vi "mqttCmdPublishTopicWrite.vi"(0 "mqttPublish in":refnum<class "mqttCmdPublish.lvclass">, 5 "topic":string, 11 "error in (no error)":errorcluster) -> (4 "mqttPublish out":refnum<class "mqttCmdPublish.lvclass">, 15 "error out":errorcluster)   [LabVIEW 2020, in "mqttCmdPublish.lvclass"]
uses:
  mqttCmdPublish.lvclass
  mqttCmdPublish.lvclass/mqttCmdPublish.ctl
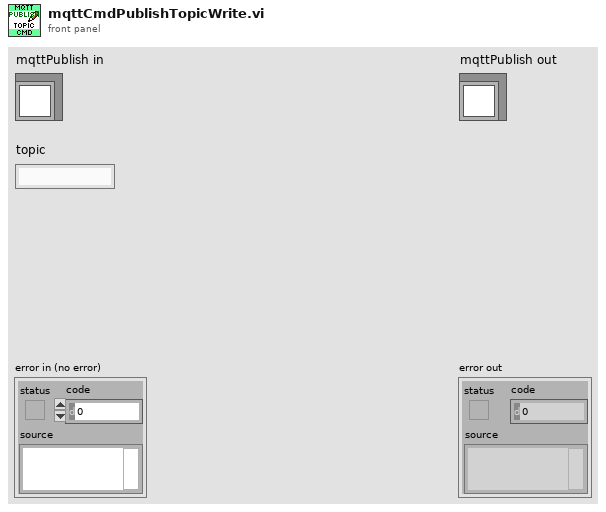
[diagram p1: front panel]
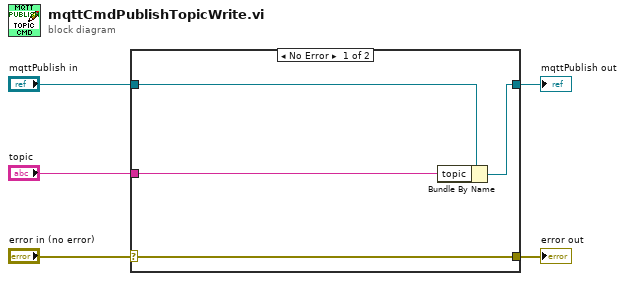
[diagram p0: block diagram]
diagram:
  n1 = case shown="No Error" "error in (no error)" {
    selector: "error in (no error)" -> [w9 w10]
    tunnel: [w9 w10] -> w4
    tunnel: [w7 w11] -> w2
    tunnel: "mqttPublish in" -> [w8 w11]
    tunnel: "topic" -> [w6 _]
    frame No Error {
      n2 = Bundle By Name(cluster=w8, "topic"=w6) -> (w7:refnum<class "mqttCmdPublish.lvclass">)
    }
    frame Error {
    }
  }
  "error out" <- w4
  "mqttPublish out" <- w2
